vi "VD-rawRequest.vi"(7 "read back?":bool, 8 "error in (no error)":errorcluster, 10 "write buffer":T1 format="%x", 11 "VD-LV-LiteVNA in":refnum<class "VD-LV-LiteVNA.lvclass">) -> (0 "error out":errorcluster, 2 "read buffer":T1 format="%x", 3 "VD-LV-LiteVNA out":refnum<class "VD-LV-LiteVNA.lvclass">)   [LabVIEW 2020, in "VD-LV-LiteVNA.lvclass"]
uses:
  VD-LV-LiteVNA.lvclass
  hardware-protocol/serial/HP-S-data.ctl
  VD-LV-LiteVNA.lvclass/VD-LV-LiteVNA.ctl
  3afb99ba-e015-4ad1-b0e7-0e458226f46f.vi
  hardware-protocol/serial/HP-S-Serial.lvclass
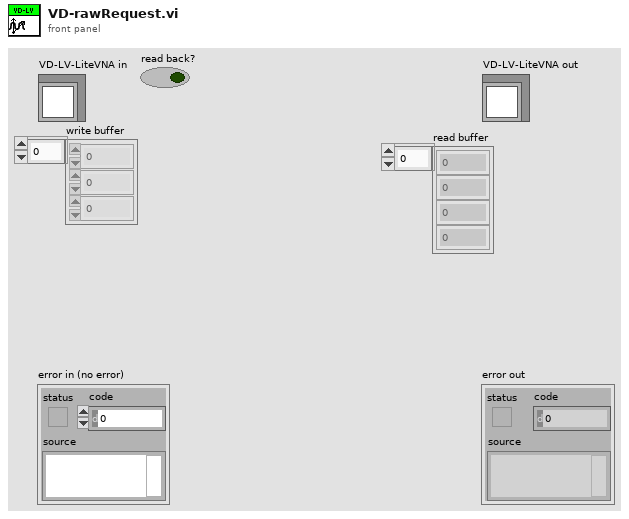
[diagram p1: front panel]
types:
  T1 = typedef "HP-S-Serial.lvclass/HP-S-data.ctl" = u8[]
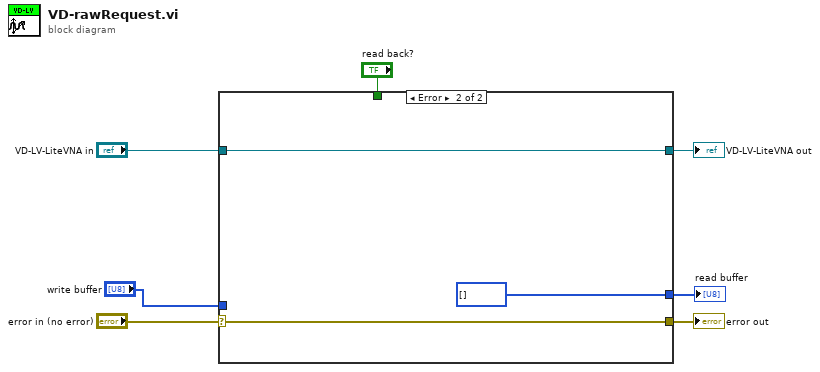
[diagram p0: block diagram]
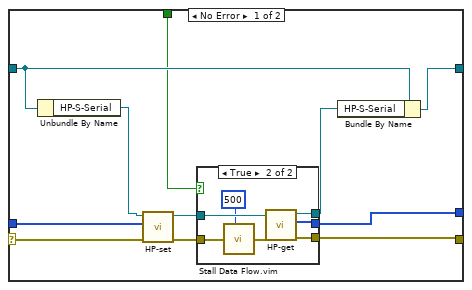
[diagram p2: hidden frame]
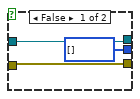
[diagram p3: hidden frame]
diagram:
  n1 = case shown="Error" "error in (no error)" {
    selector: "error in (no error)" -> [w14 w31]
    tunnel: [w11 w31] -> w6
    tunnel: [w17 w30] -> w4
    tunnel: "VD-LV-LiteVNA in" -> [w18 w30]
    tunnel: "write buffer" -> [w15 _]
    tunnel: [w10 T1 [] ("read buffer")] -> w2
    tunnel: "read back?" -> [w8 _]
    frame No Error {
      n2 = Unbundle By Name(w18) -> ("HP-S-Serial"=w16:refnum<class "HP-S-Serial.lvclass">)
      n3 = call-dynamic "HP-set.vi"("error in (no error)"=w14, "write buffer"=w15, "HP-S-Serial in"=w16) -> ("error out"=w12:errorcluster, "HP-S-Serial out"=w13:refnum<class "HP-S-Serial.lvclass">)  [unwired: 7 in]
      n4 = case shown="True" w8 {
        tunnel: w13 -> [w21 w28]
        tunnel: w12 -> [w20 w27]
        tunnel: [w20 w26] -> w11
        tunnel: [T1 [] ("read buffer") w25] -> w10
        tunnel: [w21 w24] -> w9
        frame False {
        }
        frame True {
          n5 = call "Stall Data Flow.vim"("value in"=w27, "milliseconds to wait"=u32 500) -> ("value out"=w23:errorcluster)  [unwired: 1 out]
          n6 = call-dynamic "HP-get.vi"("error in (no error)"=w23, "HP-S-Serial in"=w28) -> ("error out"=w26:errorcluster, "read buffer"=w25:T1, "HP-S-Serial out"=w24:refnum<class "HP-S-Serial.lvclass">)  [unwired: 7 in]
        }
      }
      n7 = Bundle By Name(cluster=w18, "HP-S-Serial"=w9) -> (w17:refnum<class "VD-LV-LiteVNA.lvclass">)
    }
    frame Error {
    }
  }
  "error out" <- w6
  "VD-LV-LiteVNA out" <- w4
  "read buffer" <- w2
